vi "CHS_Vision_Globals.vi"() -> ()   [LabVIEW 2019]
uses:
  <vilib>/Rock Robotics/WPI/ThirdParty/JAS_Junk/TrajLib/TypeDef/POSE2D.ctl
  <vilib>/Rock Robotics/WPI/ThirdParty/JAS_Junk/TrajLib/TypeDef/TRANSLATION2D.ctl
  <vilib>/Rock Robotics/WPI/ThirdParty/JAS_Junk/TrajLib/TypeDef/ROTATION2D.ctl
  <vilib>/Rock Robotics/WPI/ThirdParty/JAS_Junk/TrajLib/Trajectory_Library.lvlib
panel:
  out "Vison Pose":T1={"TRANSLATION"={"X"=0.0, "Y"=0.0}, "ROTATION"={"VALUE"=0.0, "COS"=1.0, "SIN"=0.0}} {"ROTATION"."SIN" format="%13.4f"; "ROTATION"."COS" format="%13.4f"; "ROTATION"."VALUE" format="%13.4f"; "TRANSLATION"."Y" format="%14.3f"; "TRANSLATION"."X" format="%14.3f"}
  out "Have Vision Pose":bool
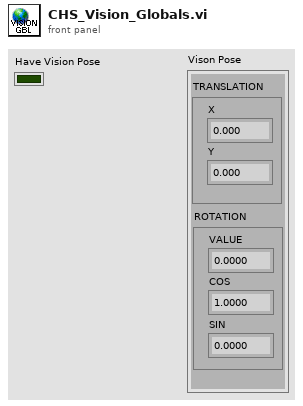
[diagram p1: front panel]
types:
  T1 = typedef "Trajectory_Library.lvlib/POSE2D.ctl" = cluster{"TRANSLATION":T2, "ROTATION":T3}
  T2 = typedef "Trajectory_Library.lvlib/TRANSLATION2D.ctl" = cluster{"X":dbl, "Y":dbl}
  T3 = typedef "Trajectory_Library.lvlib/ROTATION2D.ctl" = cluster{"VALUE":dbl, "COS":dbl, "SIN":dbl}
diagram:
